vi "ConcatenateSweepResults.vi"(8 "error in (no error)":errorcluster, 9 "SweepResults [i]":T1, 10 "SweepResults []":T1, 11 "LockinDAQ in":refnum<class "LockinDAQ.lvclass">) -> (0 "error out":errorcluster, 2 "SweepResults [] out":T1, 3 "LockinDAQ out":refnum<class "LockinDAQ.lvclass">)   [LabVIEW 2016, in "LockinDAQ.lvclass"]
uses:
  LockinDAQ.lvclass
  Typedefs/SweepResults--Cluster.ctl
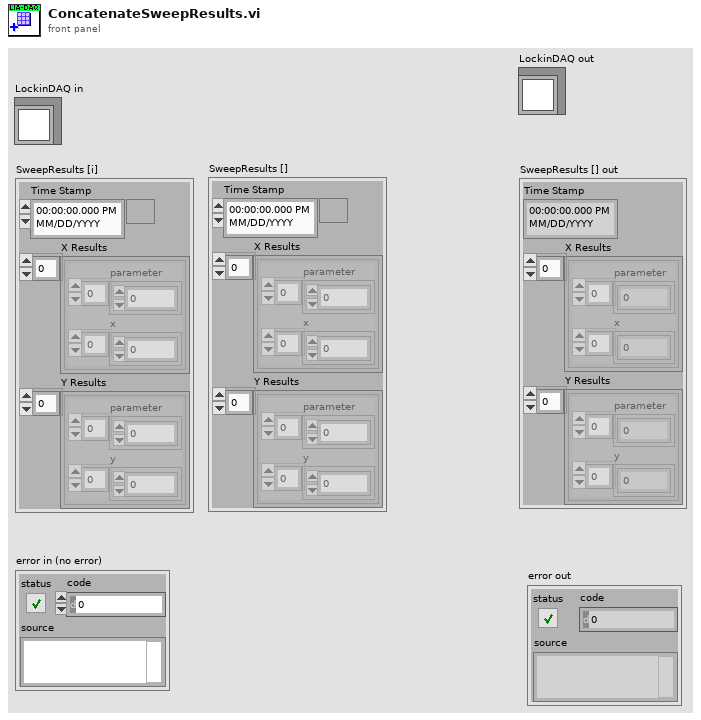
[diagram p1: front panel]
types:
  T1 = typedef "LockinDAQ.lvclass/SweepResults--Cluster.ctl" = cluster{"Time Stamp":timestamp, "X Results":cluster{"parameter":dbl[], "x":dbl[]}[], "Y Results":cluster{"parameter":dbl[], "y":dbl[]}[]}
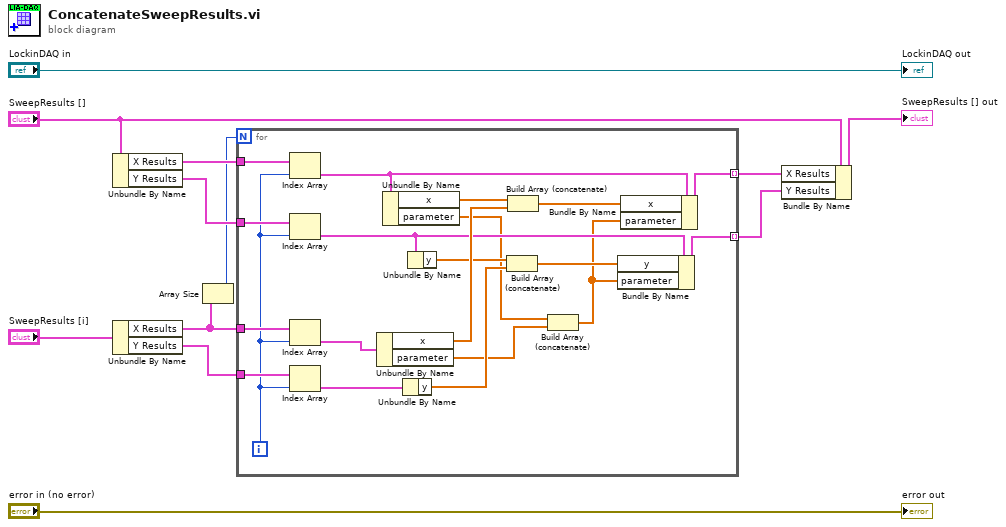
[diagram p0: block diagram]
diagram:
  n1 = Unbundle By Name("SweepResults []") -> ("X Results"=w10:cluster{"parameter":dbl[], "x":dbl[]}[], "Y Results"=w9:cluster{"parameter":dbl[], "y":dbl[]}[])
  n2 = Unbundle By Name("SweepResults [i]") -> ("X Results"=w8:cluster{"parameter":dbl[], "x":dbl[]}[], "Y Results"=w11:cluster{"parameter":dbl[], "y":dbl[]}[])
  n3 = Array Size(array=w8) -> (size(s)=w7:i32)
  n4 = for {
    N: w7 -> [_]
    tunnel: [w32] -> w5 mode=indexing
    tunnel: w8 -> [w30]
    tunnel: w11 -> [w29]
    tunnel: w10 -> [w31]
    tunnel: w9 -> [w28]
    tunnel: [w17] -> w4 mode=indexing
    i -> [w27]
    n5 = Index Array(array=w31, index=w27) -> (element=w16:cluster{"parameter":dbl[], "x":dbl[]})
    n6 = Index Array(array=w28, index=w27) -> (element=w21:cluster{"parameter":dbl[], "y":dbl[]})
    n7 = Index Array(array=w30, index=w27) -> (element=w26:cluster{"parameter":dbl[], "x":dbl[]})
    n8 = Index Array(array=w29, index=w27) -> (element=w25:cluster{"parameter":dbl[], "y":dbl[]})
    n9 = Unbundle By Name(w26) -> ("x"=w23:dbl[], "parameter"=w15:dbl[])
    n10 = Unbundle By Name(w16) -> ("x"=w24:dbl[], "parameter"=w14:dbl[])
    n11 = Unbundle By Name(w25) -> ("y"=w19:dbl[])
    n12 = Unbundle By Name(w21) -> ("y"=w20:dbl[])
    n13 = Build Array (concatenate)(w20, w19) -> (w18:dbl[])
    n14 = Build Array (concatenate)(w24, w23) -> (w22:dbl[])
    n15 = Build Array (concatenate)(w14, w15) -> (w13:dbl[])
    n16 = Bundle By Name(cluster=w21, "y"=w18, "parameter"=w13) -> (w17:cluster{"parameter":dbl[], "y":dbl[]})
    n17 = Bundle By Name(cluster=w16, "x"=w22, "parameter"=w13) -> (w32:cluster{"parameter":dbl[], "x":dbl[]})
  }
  n18 = Bundle By Name(cluster="SweepResults []", "X Results"=w5, "Y Results"=w4) -> (→"SweepResults [] out":T1)
  "LockinDAQ out" <- "LockinDAQ in"
  "error out" <- "error in (no error)"
